vi "DER Info Data from INI.vi"(8 "error in":errorcluster, 11 "Config Refnum in":T3) -> (0 "error out":errorcluster, 3 "Config Refnum out":T3, 4 "DER_Info":T1)   [LabVIEW 2018, in "AE75TX Actor.lvlib" / "AE75TX.lvclass"]
uses:
  AE75TX.lvclass
  <vilib>/Utility/config.llb/Config Data RefNum.ctl
  <vilib>/ORNL/CSEISMIC DDS/CSEISMIC DDS Base/Data Types/DER_Info.ctl
  <vilib>/ORNL/CSEISMIC DDS/CSEISMIC DDS Base/Data Types/Controls/DeviceID.ctl
  <vilib>/Utility/config.llb/Read Key (String).vi
  <vilib>/Utility/config.llb/Read Key (U32).vi
  <vilib>/Utility/config.llb/Read Key (Double).vi
  <vilib>/Utility/config.llb/Read Key (Boolean).vi
  <vilib>/Utility/config.llb/NI_LVConfig.lvlib
  <vilib>/ORNL/CSEISMIC DDS/CSEISMIC DDS Base/CSEISMIC DDS.lvclass
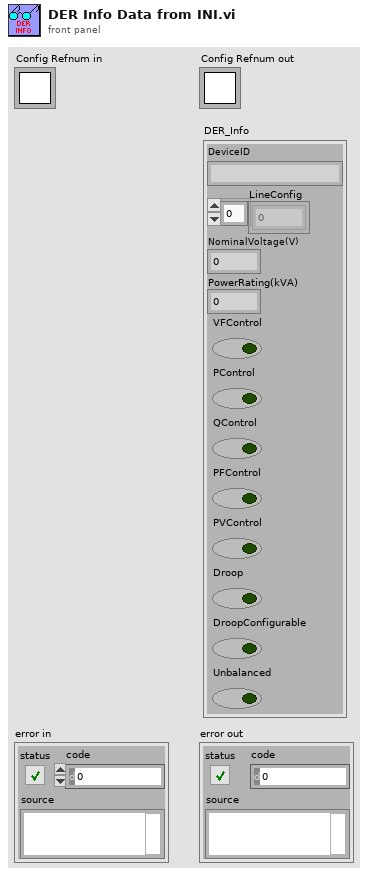
[diagram p1: front panel]
types:
  T1 = typedef "CSEISMIC DDS.lvlib/CSEISMIC DDS.lvclass/DER_Info.ctl" = cluster{"DeviceID":T2, "LineConfig":u8[], "NominalVoltage(V)":dbl, "PowerRating(kVA)":dbl, "VFControl":bool, "PControl":bool, "QControl":bool, "PFControl":bool, "PVControl":bool, "Droop":bool, "DroopConfigurable":bool, "Unbalanced":bool}
  T2 = typedef "CSEISMIC DDS.lvlib/CSEISMIC DDS.lvclass/DeviceID.ctl" = string
  T3 = typedef "NI_LVConfig.lvlib/Config Data RefNum.ctl" = refnum<k1>
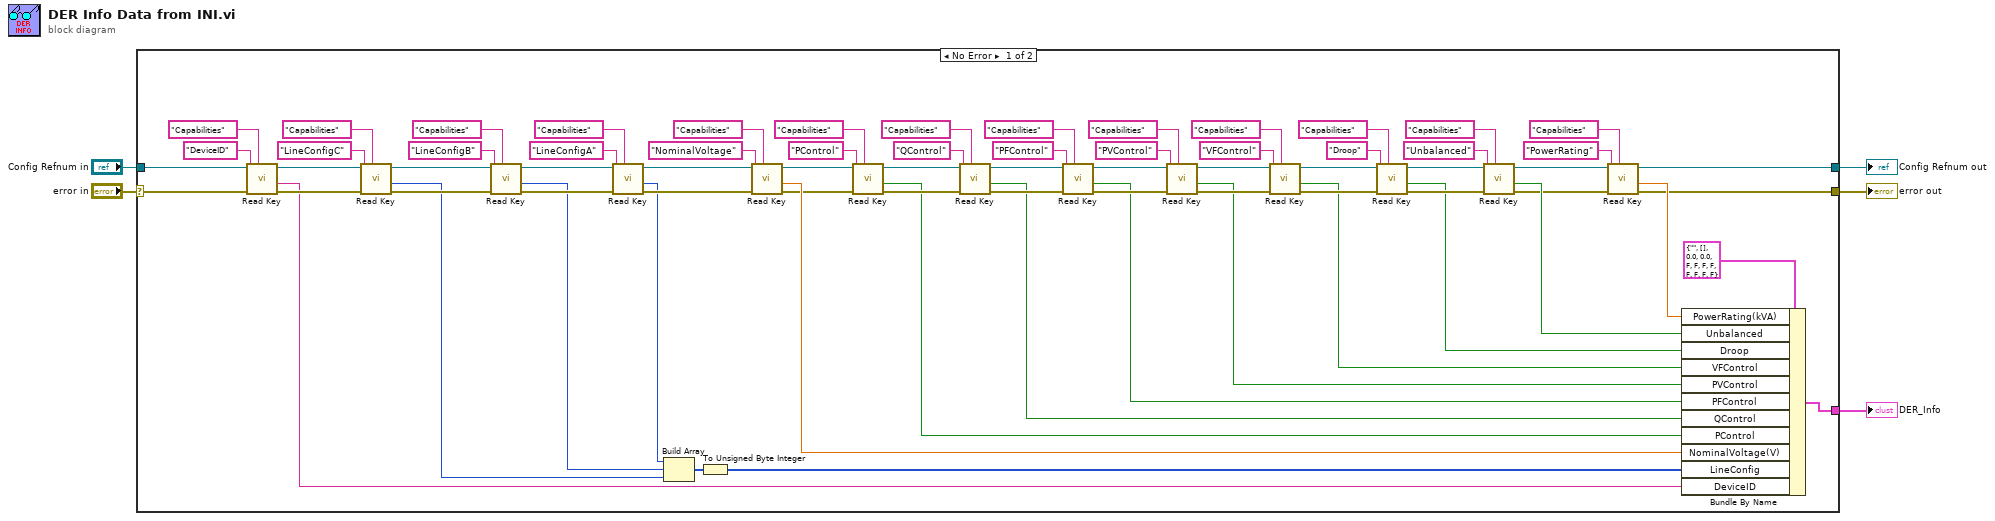
[diagram p0: block diagram]
diagram:
  n1 = case shown="No Error" "error in" {
    selector: "error in" -> [w72 w78]
    tunnel: [w7 w78] -> w5
    tunnel: [w6 w77] -> w4
    tunnel: [w76 _] -> w1
    tunnel: "Config Refnum in" -> [w73 w77]
    frame No Error {
      n2 = call-poly <vilib>:"Read Key.vi"("section"="Capabilities", "error in (no error)"=w72, "key"="DeviceID", "refnum"=w73) -> ("error out"=w60:errorcluster, "value"=w55:string, "refnum out"=w52:T3)  [unwired: 4 in, 1 out]
      n3 = call-poly <vilib>:"Read Key.vi"("section"="Capabilities", "error in (no error)"=w60, "key"="LineConfigC", "refnum"=w52) -> ("error out"=w68:errorcluster, "value"=w13:u32, "refnum out"=w67:T3)  [unwired: 4 in, 1 out]
      n4 = call-poly <vilib>:"Read Key.vi"("section"="Capabilities", "error in (no error)"=w68, "key"="LineConfigB", "refnum"=w67) -> ("error out"=w70:errorcluster, "value"=w14:u32, "refnum out"=w69:T3)  [unwired: 4 in, 1 out]
      n5 = call-poly <vilib>:"Read Key.vi"("section"="Capabilities", "error in (no error)"=w70, "key"="LineConfigA", "refnum"=w69) -> ("error out"=w56:errorcluster, "value"=w15:u32, "refnum out"=w57:T3)  [unwired: 4 in, 1 out]
      n6 = Build Array(w15, w14, w13) -> (w71:u32[])
      n7 = To Unsigned Byte Integer(number=w71) -> (unsigned 8bit integer=w54:u8[])
      n8 = call-poly <vilib>:"Read Key.vi"("section"="Capabilities", "error in (no error)"=w56, "key"="NominalVoltage", "refnum"=w57) -> ("error out"=w47:errorcluster, "value"=w53:dbl, "refnum out"=w48:T3)  [unwired: 4 in, 1 out]
      n9 = call-poly <vilib>:"Read Key.vi"("section"="Capabilities", "error in (no error)"=w47, "key"="PControl", "refnum"=w48) -> ("error out"=w37:errorcluster, "value"=w22:bool, "refnum out"=w38:T3)  [unwired: 4 in, 1 out]
      n10 = call-poly <vilib>:"Read Key.vi"("section"="Capabilities", "error in (no error)"=w37, "key"="QControl", "refnum"=w38) -> ("error out"=w36:errorcluster, "value"=w21:bool, "refnum out"=w31:T3)  [unwired: 4 in, 1 out]
      n11 = call-poly <vilib>:"Read Key.vi"("section"="Capabilities", "error in (no error)"=w36, "key"="PFControl", "refnum"=w31) -> ("error out"=w35:errorcluster, "value"=w20:bool, "refnum out"=w32:T3)  [unwired: 4 in, 1 out]
      n12 = call-poly <vilib>:"Read Key.vi"("section"="Capabilities", "error in (no error)"=w35, "key"="PVControl", "refnum"=w32) -> ("error out"=w34:errorcluster, "value"=w19:bool, "refnum out"=w33:T3)  [unwired: 4 in, 1 out]
      n13 = call-poly <vilib>:"Read Key.vi"("section"="Capabilities", "error in (no error)"=w34, "key"="VFControl", "refnum"=w33) -> ("error out"=w23:errorcluster, "value"=w18:bool, "refnum out"=w26:T3)  [unwired: 4 in, 1 out]
      n14 = call-poly <vilib>:"Read Key.vi"("section"="Capabilities", "error in (no error)"=w23, "key"="Droop", "refnum"=w26) -> ("error out"=w24:errorcluster, "value"=w17:bool, "refnum out"=w25:T3)  [unwired: 4 in, 1 out]
      n15 = call-poly <vilib>:"Read Key.vi"("section"="Capabilities", "error in (no error)"=w24, "key"="Unbalanced", "refnum"=w25) -> ("error out"=w9:errorcluster, "value"=w16:bool, "refnum out"=w10:T3)  [unwired: 4 in, 1 out]
      n16 = call-poly <vilib>:"Read Key.vi"("section"="Capabilities", "error in (no error)"=w9, "key"="PowerRating", "refnum"=w10) -> ("error out"=w7:errorcluster, "value"=w8:dbl, "refnum out"=w6:T3)  [unwired: 4 in, 1 out]
      n17 = Bundle By Name(cluster=T1 {"DeviceID"="", "LineConfig"=[], "NominalVoltage(V)"=0.0, "PowerRating(kVA)"=0.0, "VFControl"=FALSE, "PControl"=FALSE, "QControl"=FALSE, "PFControl"=FALSE, "PVControl"=FALSE, "Droop"=FALSE, "DroopConfigurable"=FALSE, "Unbalanced"=FALSE} ("DER_Info"), "PowerRating(kVA)"=w8, "Unbalanced"=w16, "Droop"=w17, "VFControl"=w18, "PVControl"=w19, "PFControl"=w20, "QControl"=w21, "PControl"=w22, "NominalVoltage(V)"=w53, "LineConfig"=w54, "DeviceID"=w55) -> (w76:T1)
    }
    frame Error {
    }
  }
  "error out" <- w5
  "Config Refnum out" <- w4
  "DER_Info" <- w1
